vi "Get DIO Port AB Bit Status.vi"(4 "error in (no error)":errorcluster, 7 "VISA resource name":refnum<visa-resource-name>) -> (0 "error out":errorcluster, 2 "DIO Port A status":T1, 3 "VISA resource name out":refnum<visa-resource-name>)   [LabVIEW 2019, in "Newport ESP301.lvlib"]
doc: "Reads all digital I/O port A,B and C logic level."
uses:
  Newport ESP301.lvlib
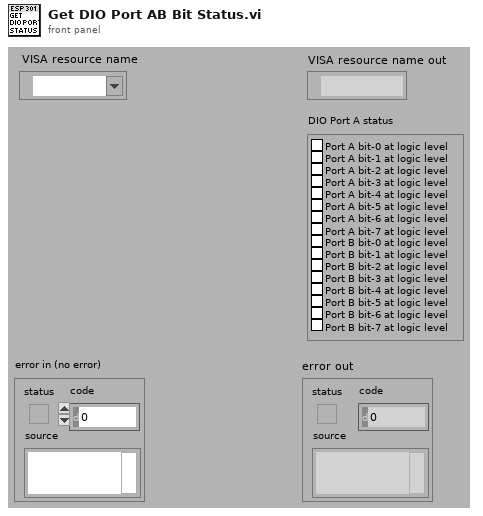
[diagram p1: front panel]
types:
  T1 = cluster{"Port A bit-0 at logic level":bool, "Port A bit-1 at logic level":bool, "Port A bit-2 at logic level ":bool, "Port A bit-3 at logic level":bool, "Port A bit-4 at logic level":bool, "Port A bit-5 at logic level ":bool, "Port A bit-6 at logic level ":bool, "Port A bit-7 at logic level ":bool, "Port B bit-0 at logic level":bool, "Port B bit-1 at logic level":bool, "Port B bit-2 at logic level ":bool, "Port B bit-3 at logic level":bool, "Port B bit-4 at logic level":bool, "Port B bit-5 at logic level ":bool, "Port B bit-6 at logic level ":bool, "Port B bit-7 at logic level ":bool}
  T2 = cluster{"Boolean array[0]":bool, "Boolean array[1]":bool, "Boolean array[2]":bool, "Boolean array[3]":bool, "Boolean array[4]":bool, "Boolean array[5]":bool, "Boolean array[6]":bool, "Boolean array[7]":bool, "Boolean array[8]":bool, "Boolean array[9]":bool, "Boolean array[10]":bool, "Boolean array[11]":bool, "Boolean array[12]":bool, "Boolean array[13]":bool, "Boolean array[14]":bool, "Boolean array[15]":bool}
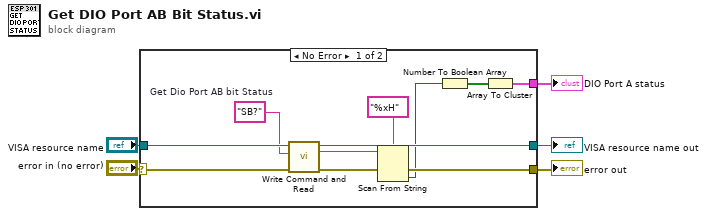
[diagram p0: block diagram]
diagram:
  n1 = case shown="No Error" "error in (no error)" {
    selector: "error in (no error)" -> [w14 w18]
    tunnel: [w10 w18] -> w5
    tunnel: "VISA resource name" -> [w16 w17]
    tunnel: [w15 w17] -> w4
    tunnel: [w7 _] -> w1
    frame No Error {
      w13 = "SB?"  # Get Dio Port AB bit Status
      n2 = call "Write Command and Read.vi"("error in (no error)"=w14, "Command"=w13, "VISA resource name"=w16) -> ("error out"=w11:errorcluster, "Returned string"=w9:string, "VISA resource name out"=w15:refnum<visa-resource-name>)  [unwired: 2 in, 2 out]
      n3 = Scan From String(format string="%xH" ("chaîne de format"), input string=w9, error in=w11) -> (error out=w10:errorcluster, output 1=w8:u32)  [unwired: 2 in, 2 out]
      n4 = Number To Boolean Array(number=w8) -> (Boolean array=w12:bool[])
      n5 = Array To Cluster(array=w12) -> (cluster=w7:T2)
    }
    frame Error {
    }
  }
  "error out" <- w5
  "VISA resource name out" <- w4
  "DIO Port A status" <- w1
